vi "lqManifestation.vi"(11 "LQSerialData in":refnum<class "LQSerialData.lvclass">) -> (2 "Manifestation":string, 3 "LQSerialData out":refnum<class "LQSerialData.lvclass">)   [LabVIEW 2013, in "Template.lvlib" / "LQSerialData.lvclass"]
uses:
  LQSerialData.lvclass
  LQSerialData.lvclass/LQSerialData.ctl
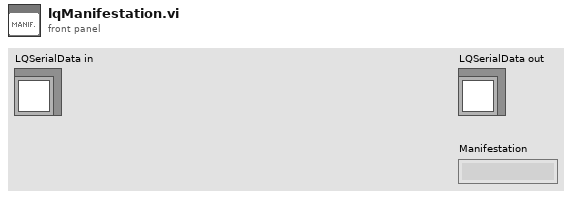
[diagram p1: front panel]
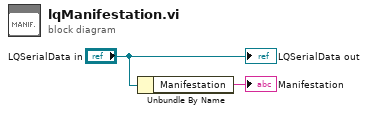
[diagram p0: block diagram]
diagram:
  n1 = Unbundle By Name("LQSerialData in") -> ("Manifestation"=→"Manifestation":string)
  "LQSerialData out" <- "LQSerialData in"
